vi "GetConnection.vi"(8 "error in (no error)":errorcluster, 11 "ClientBase in":refnum<class "ClientBase.lvclass">) -> (0 "error out":errorcluster, 2 "connection ID":refnum<k5>, 3 "ClientBase out":refnum<class "ClientBase.lvclass">)   [LabVIEW 2020, in "ClientBaseLib.lvlib" / "ClientBase.lvclass"]
uses:
  ClientBase.lvclass
  ClientBase.lvclass/ClientBase.ctl
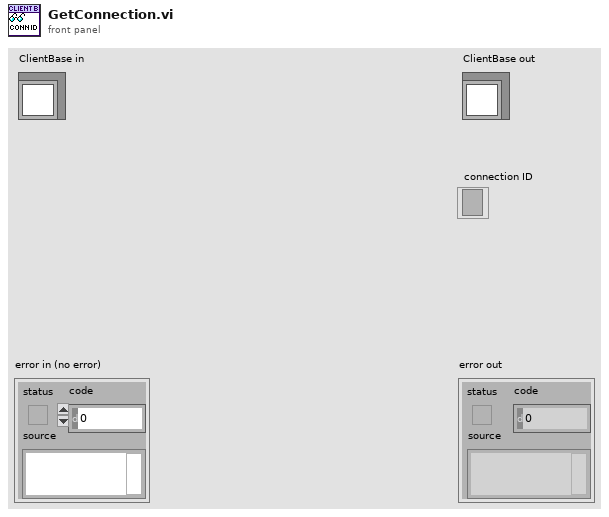
[diagram p1: front panel]
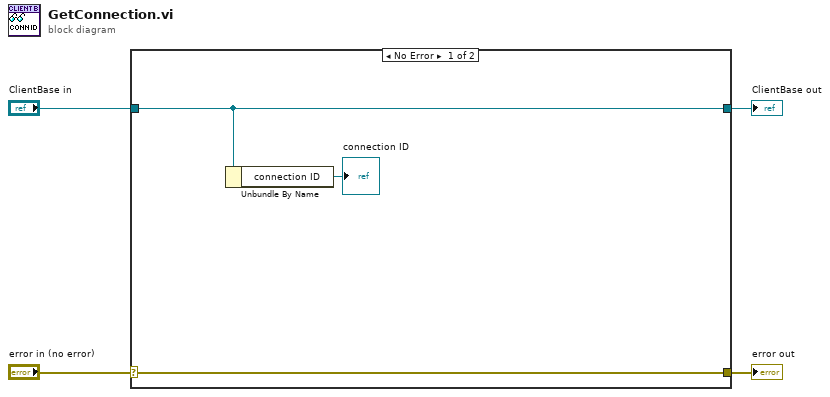
[diagram p0: block diagram]
diagram:
  n1 = case shown="No Error" "error in (no error)" {
    selector: "error in (no error)" -> [w7 w9]
    tunnel: [w7 w9] -> w3
    tunnel: [w6 w8] -> w1
    tunnel: "ClientBase in" -> [w6 w8]
    frame No Error {
      n2 = Unbundle By Name(w6) -> ("connection ID"=→"connection ID":refnum<k5>)
    }
    frame Error {
    }
  }
  "error out" <- w3
  "ClientBase out" <- w1
